vi "acquisition.vi"(8 "Erreur en entrée":errorcluster, 11 "ID d'entrée":T1) -> (0 "sortie d'erreur":errorcluster, 2 "Graphe de l'entrée":cluster{"Numeric":dbl, dbl}, 3 "ID de sortie":T1, 5 "sortie avant":dbl, 7 "sortie arriere":dbl)   [LabVIEW 2019]
uses:
  <instrlib>/Sefram DAS240/Sefram DAS240.lvlib
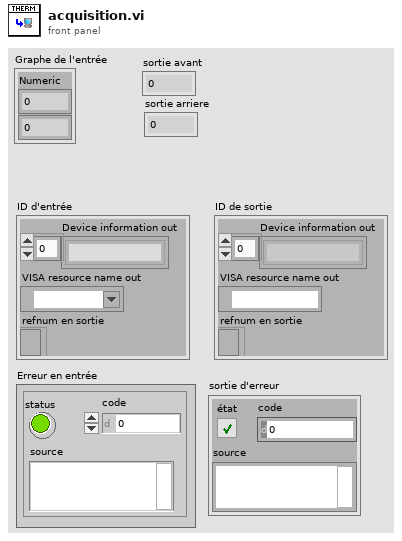
[diagram p1: front panel]
types:
  T1 = cluster{"Device information out":string[], "VISA resource name out":refnum<visa-resource-name>, "refnum en sortie":refnum<file>}
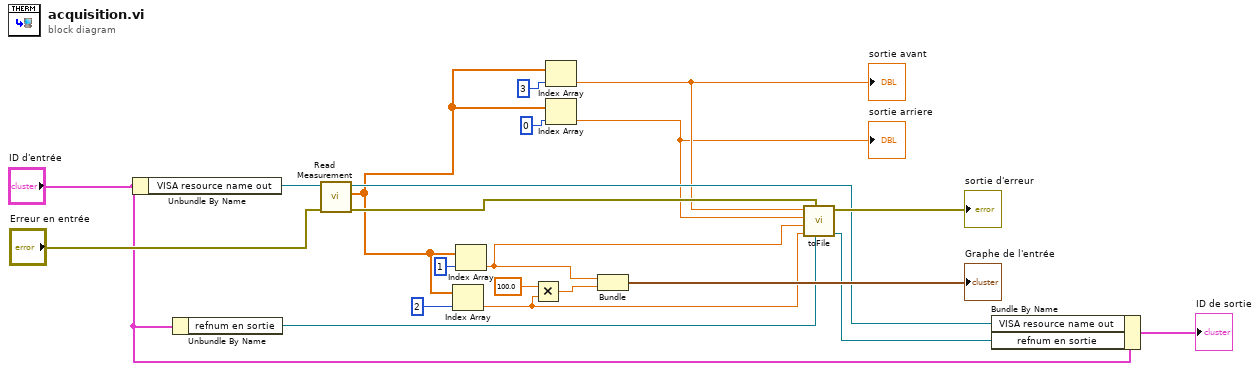
[diagram p0: block diagram]
diagram:
  n1 = Unbundle By Name("ID d'entrée") -> ("VISA resource name out"=w13:refnum<visa-resource-name>)
  n2 = Unbundle By Name("ID d'entrée") -> ("refnum en sortie"=w11:refnum<file>)
  n3 = call <instrlib>:"Read Measurement.vi"("error in (no error)"="Erreur en entrée", "VISA resource name"=w13) -> ("error out"=w4:errorcluster, "Data"=w2:dbl[], "VISA resource name out"=w7:refnum<visa-resource-name>)  [unwired: 7 in]
  n4 = Index Array(array=w2, index=2 ("indice")) -> (element=w16:dbl)
  n5 = Index Array(array=w2, index=1 ("indice")) -> (element=w18:dbl)
  n6 = Multiply(x=100.0, y=w16) -> (x*y=w14:dbl)
  n7 = Index Array(array=w2, index=3 ("indice")) -> (element=w3:dbl)
  "sortie avant" <- w3
  n8 = Index Array(array=w2, index=0 ("indice")) -> (element=w1:dbl)
  "sortie arriere" <- w1
  n9 = Bundle("Numeric"=w18, w14) -> (→"Graphe de l'entrée":cluster{"Numeric":dbl, dbl})  [unwired: 1 in]
  n10 = call "toFile.vi"("refnum"=w11, "entrée d'erreur"=w4, "entree V"=w16, "entree phi"=w18, "sortie arr"=w1, "sortie avant"=w3) -> ("refnum en sortie"=w8:refnum<file>, "sortie d'erreur"=→"sortie d'erreur":errorcluster)  [unwired: 4 in]
  n11 = Bundle By Name(cluster="ID d'entrée", "VISA resource name out"=w7, "refnum en sortie"=w8) -> (→"ID de sortie":T1)
